vi "Parse-attributes.vi"(8 "error in (no error)":errorcluster, 10 "String in":string, 11 "Element-XML in":refnum<class "Element-XML.lvclass">) -> (0 "error out":errorcluster, 1 "Valid attributes?":bool, 2 "Remaining string":string, 3 "Element-XML out":refnum<class "Element-XML.lvclass">, 4 "Remaining content?":bool)   [LabVIEW 2013, in "MaterialCharacterization.lvlib" / "Element-XML.lvclass"]
uses:
  Element-XML.lvclass
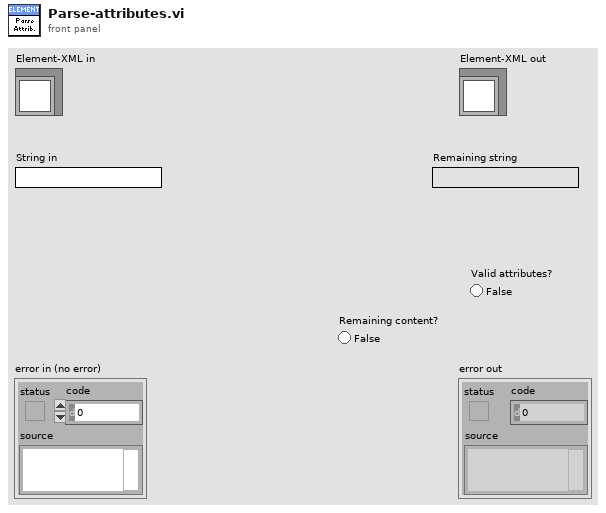
[diagram p1: front panel]
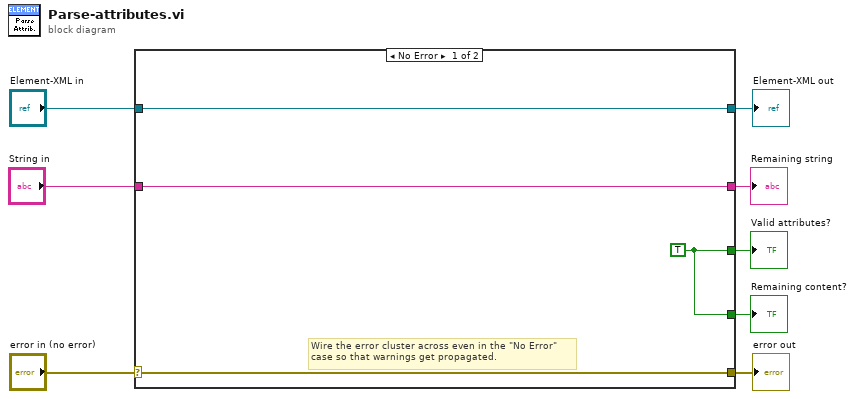
[diagram p0: block diagram]
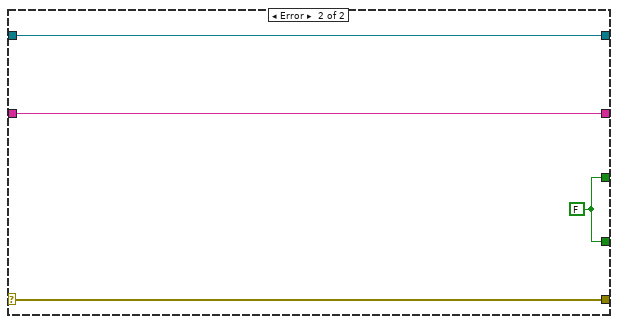
[diagram p2: hidden frame]
diagram:
  n1 = case shown="No Error" "error in (no error)" {
    selector: "error in (no error)" -> [w11 w16]
    tunnel: [w11 w16] -> w7
    tunnel: [w12 w15] -> w5
    tunnel: "Element-XML in" -> [w12 w15]
    tunnel: "String in" -> [w10 w14]
    tunnel: [w10 w14] -> w3
    tunnel: [w9 w13] -> w2
    tunnel: [w9 w13] -> w1
    frame No Error {
      w9 = TRUE
      # "Wire the error cluster across even in the \"No Error\"\ncase so that warnings get propagated."
    }
    frame Error {
      w13 = FALSE
    }
  }
  "error out" <- w7
  "Element-XML out" <- w5
  "Valid attributes?" <- w2
  "Remaining string" <- w3
  "Remaining content?" <- w1
